vi "Set simulated or real mode.vi"(8 "error in (no error)":errorcluster, 11 "Channel in":refnum<class "Channel.lvclass">) -> (0 "error out":errorcluster, 3 "Channel out":refnum<class "Channel.lvclass">)   [LabVIEW 2018, in "Channel.lvclass"]
doc: "Choose between the simulated or real camera class"
uses:
  Channel.lvclass
  CCDCamera/CCDCamera.lvclass
  C:/Users/observer/Desktop/SPARC4_ACS/SPARC4_ACS/Simulated_CCD_Camera/Simulated_CCD_Camera.lvclass
  Channel.lvclass/Channel.ctl
panel:
  in  "CCDCamera.lvclass":refnum<class "CCDCamera.lvclass">
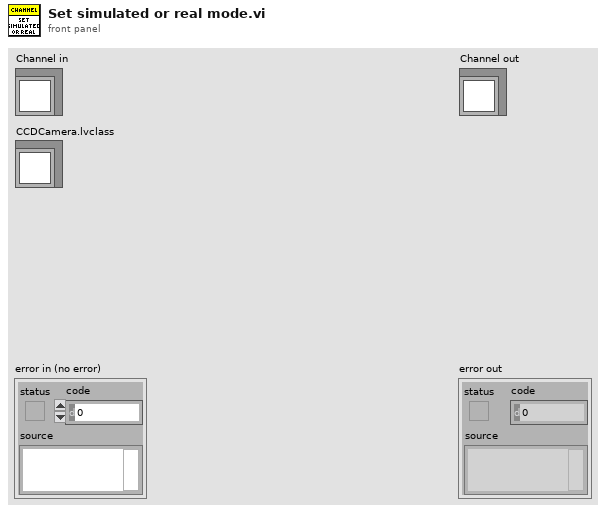
[diagram p1: front panel]
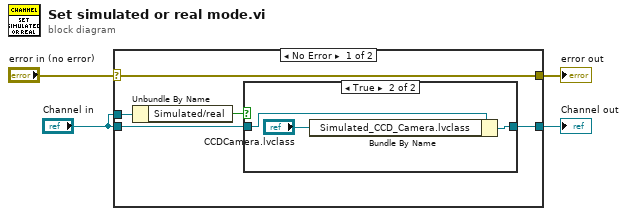
[diagram p0: block diagram]
diagram:
  n1 = case shown="No Error" "error in (no error)" {
    selector: "error in (no error)" -> [w7 w15]
    tunnel: [w7 w15] -> w3
    tunnel: [w5 w14] -> w2
    tunnel: "Channel in" -> [w8 w14]
    tunnel: "Channel in" -> [w6 _]
    frame No Error {
      n2 = Unbundle By Name(w8) -> ("Simulated/real"=w9:bool)
      n3 = case shown="True" w9 {
        tunnel: w6 -> [w10 w13]
        tunnel: [w10 w11] -> w5
        frame False {
        }
        frame True {
          n4 = Bundle By Name(cluster=w13, "Simulated_CCD_Camera.lvclass"="CCDCamera.lvclass") -> (w11:refnum<class "Channel.lvclass">)
        }
      }
    }
    frame Error {
    }
  }
  "error out" <- w3
  "Channel out" <- w2
